vi "Format Number.vi"(5 "Data":T1, 7 "precision (6)":i16, 9 "Format":T2 items=["Decimal"=0, "Scientific"=1, "Hexadecimal"=5]) -> (8 "Numeric String":string)   [LabVIEW 2013, in "Calculator XControl.xctl"]
uses:
  Calculator XControl.xctl
  Controls/Format.ctl
  Core/Data.ctl
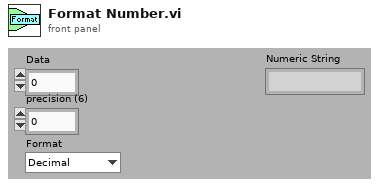
[diagram p1: front panel]
types:
  T1 = typedef "Calculator XControl.xctl/Data.ctl" = dbl
  T2 = typedef "Calculator XControl.xctl/Format.ctl" = u16
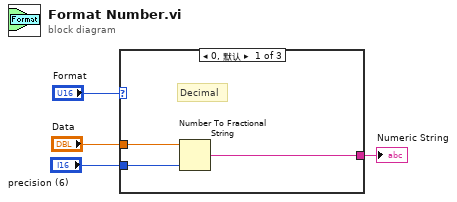
[diagram p0: block diagram]
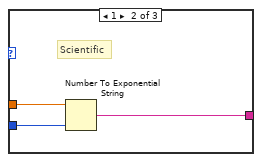
[diagram p2: hidden frame]
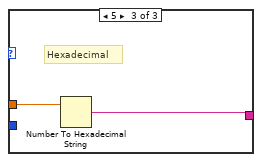
[diagram p3: hidden frame]
diagram:
  n1 = case shown="0, 默认" "Format" {
    tunnel: "Data" -> [w7 w10 w12]
    tunnel: [w6 w8 w11] -> w2
    tunnel: "precision (6)" -> [w5 w9 _]
    frame 0, Default {
      # "Decimal"
      n2 = Number To Fractional String(number=w7, precision (6)=w5) -> (F-format string=w6:string)  [unwired: 2 in]
    }
    frame 1 {
      # "Scientific"
      n3 = Number To Exponential String(number=w10, precision (6)=w9) -> (E-format string=w8:string)  [unwired: 2 in]
    }
    frame 5 {
      # "Hexadecimal"
      n4 = Number To Hexadecimal String(2:w12) -> (0:w11:string)  [unwired: 1 in]
    }
  }
  "Numeric String" <- w2
